vi "encoder read.vi"(1 "Reset M1":bool, 2 "Reset M2":bool, 3 "Reset M3":bool, 4 "Reset  All":bool, 5 "handle":i32) -> (9 "M1-Encoder (um)":dbl format="%.3f", 11 "M2-Encoder (um)":dbl format="%.3f", 13 "M3-Encoder (um)":dbl format="%.3f", 14 "M1 Reverse Limit":bool, 15 "M1 Forward Limit":bool, 16 "M2 Reverse Limit":bool, 17 "M2 Forward Limit":bool, 18 "M3 Reverse Limit":bool, 19 "M3 Forward Limit":bool)   [LabVIEW 2020]
uses:
  MicroDrive.dll
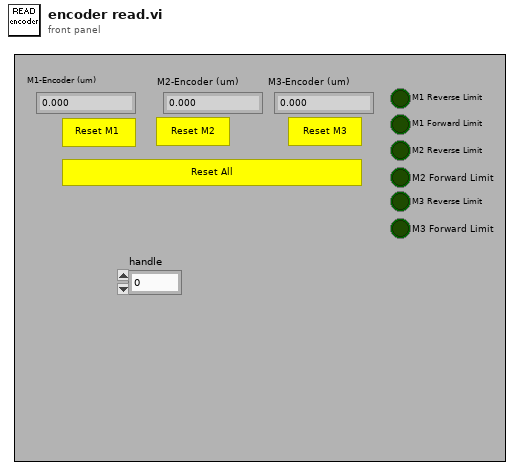
[diagram p1: front panel]
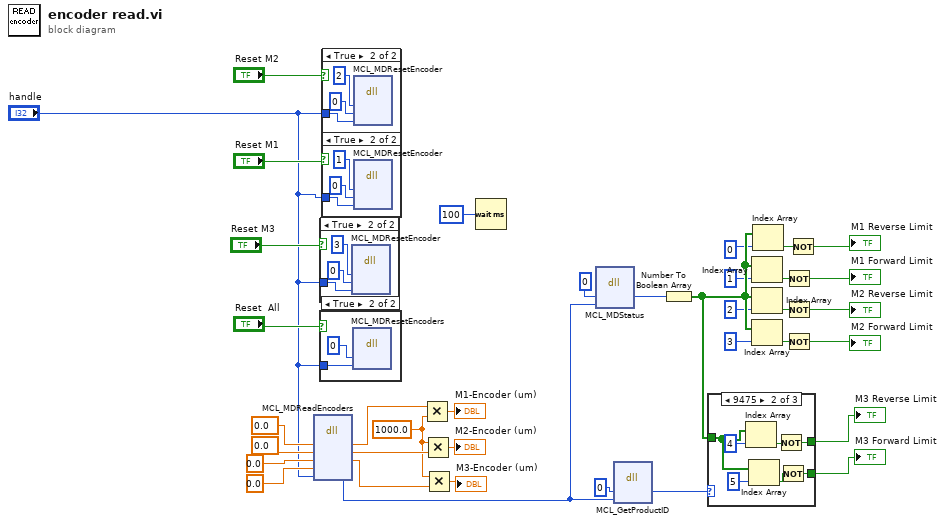
[diagram p0: block diagram]
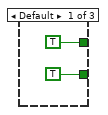
[diagram p4: hidden frame]
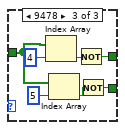
[diagram p5: hidden frame]
diagram:
  w25 = 1000.0
  n1 = dll-call lib="C:/Users/WalsworthGroup/Documents/Mad City Labs/MicroDrive/Labview Examples/MicroDrive.dll" fn="MCL_MDReadEncoders"("e1"=0.0, "e2"=0.0, "e3"=0.0 ("zenc"), "e4"=0.0 ("zenc"), "handle"="handle") -> ("e1"=w34:dbl, "e2"=w33:dbl, "e3"=w26:dbl, "handle"=w8:i32)  [unwired: 3 in, 4 out]
  n2 = case shown="True" "Reset M3" {
    tunnel: "handle" -> [_ w40]
    frame False {
    }
    frame True {
      n3 = dll-call lib="C:/Users/WalsworthGroup/Documents/Mad City Labs/MicroDrive/Labview Examples/MicroDrive.dll" fn="MCL_MDResetEncoder"("axis"=u32 3, "status"=u16 0, "handle"=w40) -> ()  [unwired: 4 in, 5 out]
    }
  }
  n4 = case shown="True" "Reset  All" {
    tunnel: "handle" -> [_ w42]
    frame False {
    }
    frame True {
      n5 = dll-call lib="C:/Users/WalsworthGroup/Documents/Mad City Labs/MicroDrive/Labview Examples/MicroDrive.dll" fn="MCL_MDResetEncoders"("status"=u16 0, "handle"=w42) -> ()  [unwired: 4 in, 4 out]
    }
  }
  n6 = case shown="True" "Reset M2" {
    tunnel: "handle" -> [_ w45]
    frame False {
    }
    frame True {
      n7 = dll-call lib="C:/Users/WalsworthGroup/Documents/Mad City Labs/MicroDrive/Labview Examples/MicroDrive.dll" fn="MCL_MDResetEncoder"("axis"=u32 2, "status"=u16 0, "handle"=w45) -> ()  [unwired: 4 in, 5 out]
    }
  }
  n8 = case shown="True" "Reset M1" {
    tunnel: "handle" -> [_ w48]
    frame False {
    }
    frame True {
      n9 = dll-call lib="C:/Users/WalsworthGroup/Documents/Mad City Labs/MicroDrive/Labview Examples/MicroDrive.dll" fn="MCL_MDResetEncoder"("axis"=u32 1, "status"=u16 0, "handle"=w48) -> ()  [unwired: 4 in, 5 out]
    }
  }
  n10 = Multiply(x=w34, y=w25) -> (x*y=→"M1-Encoder (um)":dbl)
  n11 = Multiply(x=w25, y=w33) -> (x*y=→"M2-Encoder (um)":dbl)
  n12 = Multiply(x=w25, y=w26) -> (x*y=→"M3-Encoder (um)":dbl)
  n13 = Wait (ms)(milliseconds to wait=100) -> ()  [unwired: 1 out]
  n14 = dll-call lib="C:/Users/WalsworthGroup/Documents/Mad City Labs/MicroDrive/Labview Examples/MicroDrive.dll" fn="MCL_MDStatus"("status"=u16 0, "handle"=w8) -> ("status"=w5:u16)  [unwired: 4 in, 3 out]
  n15 = dll-call lib="C:/Users/WalsworthGroup/Documents/Mad City Labs/MicroDrive/Labview Examples/MicroDrive.dll" fn="MCL_GetProductID"("PID"=u16 0, "handle"=w8) -> ("PID"=w21:u16)  [unwired: 4 in, 3 out]
  n16 = Number To Boolean Array(number=w5) -> (Boolean array=w22:bool[])
  n17 = case shown="9475" w21 {
    tunnel: w22 -> [_ w57 w58]
    tunnel: [TRUE w53 w60] -> w23
    tunnel: [TRUE w51 w59] -> w24
    frame Default {
    }
    frame 9475 {
      n18 = Index Array(array=w57, index=4) -> (element=w52:bool)
      n19 = Index Array(array=w57, index=5) -> (element=w54:bool)
      n20 = Not(x=w52) -> (.not. x?=w51:bool)
      n21 = Not(x=w54) -> (.not. x?=w53:bool)
    }
    frame 9478 {
      n22 = Index Array(array=w58, index=4) -> (element=w61:bool)
      n23 = Index Array(array=w58, index=5) -> (element=w62:bool)
      n24 = Not(x=w61) -> (.not. x?=w59:bool)
      n25 = Not(x=w62) -> (.not. x?=w60:bool)
    }
  }
  "M3 Reverse Limit" <- w24
  "M3 Forward Limit" <- w23
  n26 = Index Array(array=w22, index=1) -> (element=w18:bool)
  n27 = Index Array(array=w22, index=2) -> (element=w17:bool)
  n28 = Index Array(array=w22, index=3) -> (element=w16:bool)
  n29 = Index Array(array=w22, index=0) -> (element=w6:bool)
  n30 = Not(x=w18) -> (.not. x?=→"M1 Forward Limit":bool)
  n31 = Not(x=w17) -> (.not. x?=→"M2 Reverse Limit":bool)
  n32 = Not(x=w16) -> (.not. x?=→"M2 Forward Limit":bool)
  n33 = Not(x=w6) -> (.not. x?=→"M1 Reverse Limit":bool)
